vi "의사결정 구조 실습.vi"() -> ()   [LabVIEW 2020]
panel:
  out "숫자형 6":i32
  in  "정지입니다.":bool
  out "숫자형 5":i32
  in  "버튼입니다.":bool
  out "숫자형 4":dbl
  in  "숫자형 3":dbl
  in  "숫자형 2":dbl
  in  "문자열":string
  in  "숫자형":i32
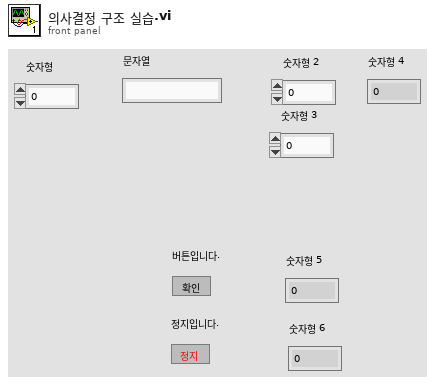
[diagram p1: front panel]
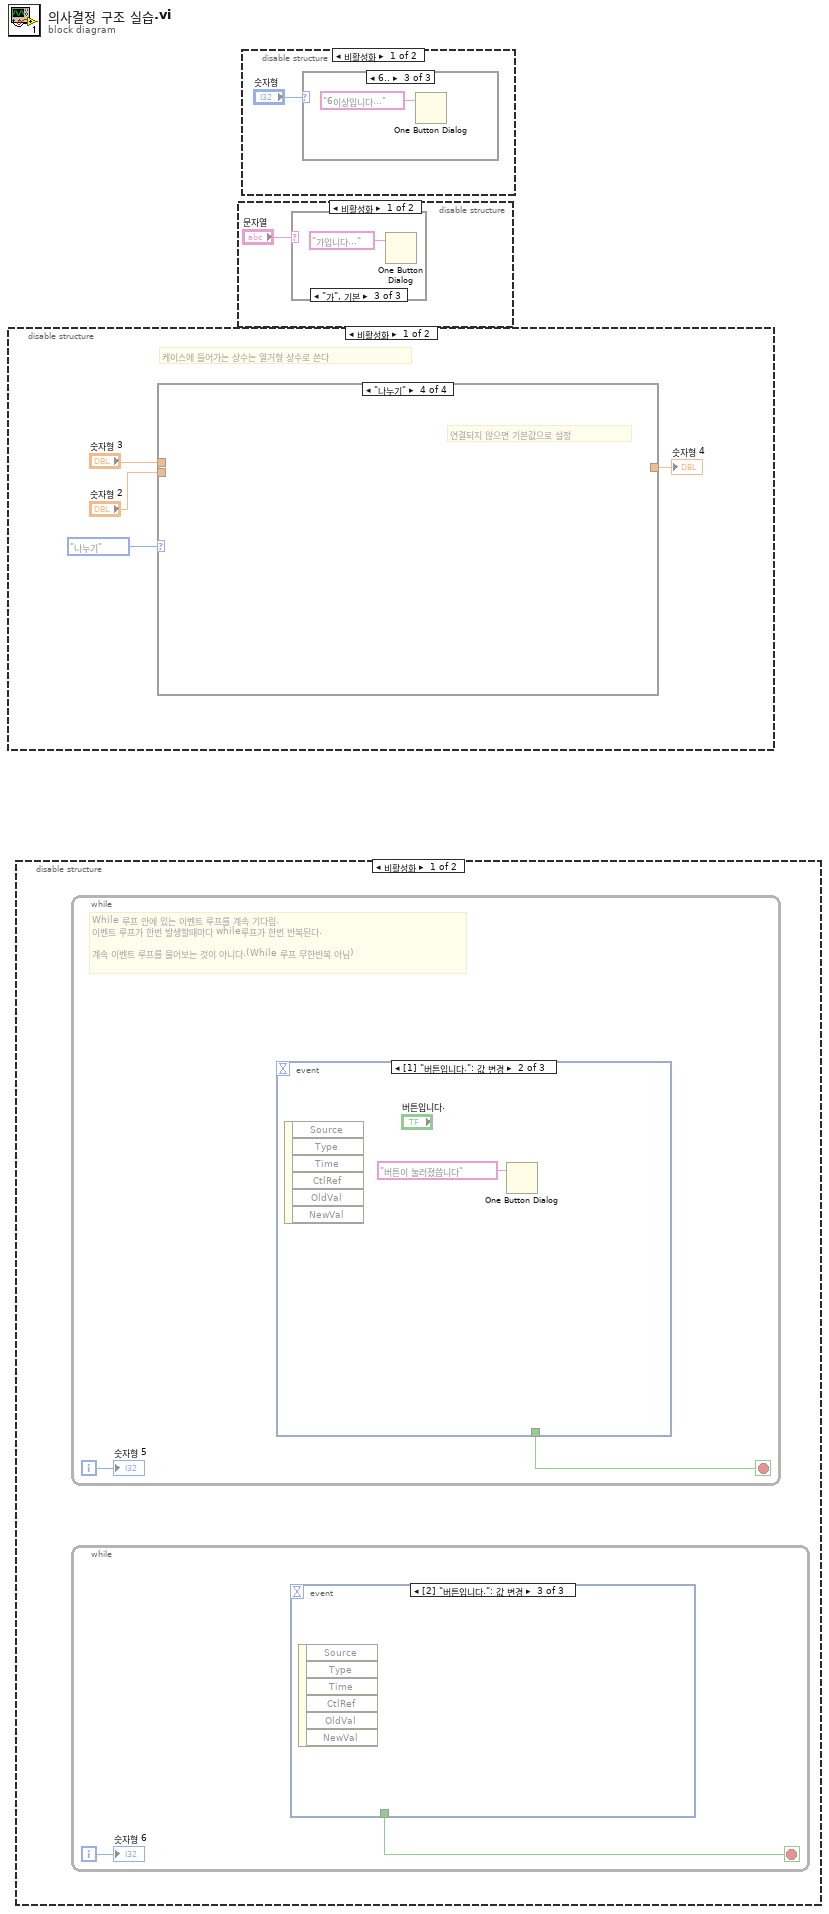
[diagram p0: block diagram]
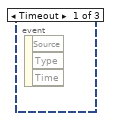
[diagram p2: hidden frame]
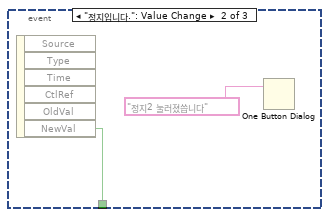
[diagram p3: hidden frame]
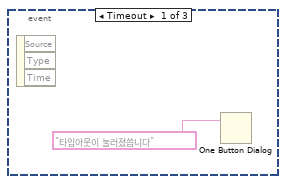
[diagram p4: hidden frame]
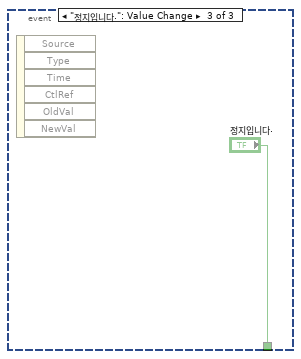
[diagram p5: hidden frame]
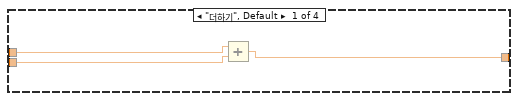
[diagram p7: hidden frame]
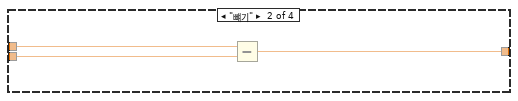
[diagram p8: hidden frame]
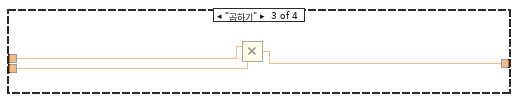
[diagram p9: hidden frame]
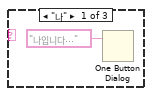
[diagram p11: hidden frame]
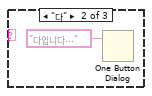
[diagram p12: hidden frame]
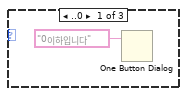
[diagram p14: hidden frame]
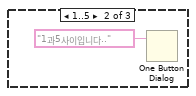
[diagram p15: hidden frame]
diagram:
  n1 = disable-structure shown="비활성화" {
    frame Disabled {
      # "케이스에 들어가는 상수는 열거형 상수로 쓴다"
      n2 = case shown="\"나누기\"" enum16{"더하기", "뺴기", "곱하기", "나누기"}."나누기" ("열거형") {
        tunnel: "숫자형 3" -> [w7 w10 w13 _]
        tunnel: "숫자형 2" -> [w6 w9 w12 _]
        tunnel: [w5 w8 w11 _] -> w1
        frame "더하기", Default {
          n3 = Add(x=w7, y=w6) -> (x+y=w5:dbl)
        }
        frame "뺴기" {
          n4 = Subtract(x=w10, y=w9) -> (x-y=w8:dbl)
        }
        frame "곱하기" {
          n5 = Multiply(x=w13, y=w12) -> (x*y=w11:dbl)
        }
        frame "나누기" {
          # "연결되지 않으면 기본값으로 설정"
        }
      }
      "숫자형 4" <- w1
    }
    frame Enabled {
    }
  }
  n6 = disable-structure shown="비활성화" {
    frame Disabled {
      n7 = while {
        i -> [w19]
        stop <- w18 stop-if-true
        # "While 루프 안에 있는 이벤트 루프를 계속 기다림.\n이벤트 루프가 한번 발생할때마다 while루프가 한번 반복된다.\n\n계속 이벤트 루프를 물어보는 것이 아니다.(While 루프 무한반복 아님)"
        n8 = event shown="[1] \"버튼입니다.\": 값 변경" {
          selector: _ -> [_ _ _]
          dyn-events: _ -> [_ _ _]
          timeout: _ -> [_ _ _]
          tunnel: [_ _ "정지입니다."] -> w18
          event Timeout {
            n9 = event-data() -> ()  [unwired: 1 in, 3 out]
            n10 = One Button Dialog(message="타임아웃이 눌러졌씁니다" ("메시지")) -> ()  [unwired: 1 in, 1 out]
          }
          event "버튼입니다.": Value Change {
            n11 = event-data() -> ()  [unwired: 1 in, 6 out]
            n12 = One Button Dialog(message="버튼이 눌러졌씁니다" ("메시지")) -> ()  [unwired: 1 in, 1 out]
          }
          event "정지입니다.": Value Change {
            n13 = event-data() -> ()  [unwired: 1 in, 6 out]
          }
        }
        "숫자형 5" <- w19
      }
      n14 = while {
        i -> [w14]
        stop <- w15 stop-if-true
        n15 = event shown="[2] \"버튼입니다.\": 값 변경" {
          selector: _ -> [_ _ _]
          dyn-events: _ -> [_ _ _]
          timeout: _ -> [_ _ _]
          tunnel: [_ w17 _] -> w15
          event Timeout {
            n16 = event-data() -> ()  [unwired: 1 in, 3 out]
          }
          event "정지입니다.": Value Change {
            n17 = event-data() -> ("NewVal"=w17:bool)  [unwired: 1 in, 5 out]
            n18 = One Button Dialog(message="정지2 눌러졌씁니다" ("메시지")) -> ()  [unwired: 1 in, 1 out]
          }
          event "버튼입니다.": Value Change {
            n19 = event-data() -> ()  [unwired: 1 in, 6 out]
          }
        }
        "숫자형 6" <- w14
      }
    }
    frame Enabled {
    }
  }
  n20 = disable-structure shown="비활성화" {
    frame Disabled {
      n21 = case shown="\"가\", 기본" "문자열" {
        frame "나" {
          n22 = One Button Dialog(message="나입니다..." ("메시지")) -> ()  [unwired: 1 in, 1 out]
        }
        frame "다" {
          n23 = One Button Dialog(message="다입니다..." ("메시지")) -> ()  [unwired: 1 in, 1 out]
        }
        frame "가", Default {
          n24 = One Button Dialog(message="가입니다..." ("메시지")) -> ()  [unwired: 1 in, 1 out]
        }
      }
    }
    frame Enabled {
    }
  }
  n25 = disable-structure shown="비활성화" {
    frame Disabled {
      n26 = case shown="6.." "숫자형" {
        frame ..0 {
          n27 = One Button Dialog(message="0이하입니다" ("메시지")) -> ()  [unwired: 1 in, 1 out]
        }
        frame 1..5 {
          n28 = One Button Dialog(message="1과5사이입니다.." ("메시지")) -> ()  [unwired: 1 in, 1 out]
        }
        frame 6.. {
          n29 = One Button Dialog(message="6이상입니다..." ("메시지")) -> ()  [unwired: 1 in, 1 out]
        }
      }
    }
    frame Enabled {
    }
  }
